vi "New Round.vi"(8 "error in (no error)":errorcluster, 10 "Move Count":i32, 11 "Grid":T1) -> (0 "error out":errorcluster, 3 "Grid out":T1)   [LabVIEW 2014, in "TeamEffort.lvclass"]
uses:
  Square/Shawn/TeamEffort/TeamEffort.lvclass
  SquareBattle Arena/Action Enum.ctl
  SquareBattle Arena/SquareBattle Arena.lvclass
  SquareBattle Arena/Direction Enum.ctl
  Player Cluster.ctl
  Grid Cluster.ctl
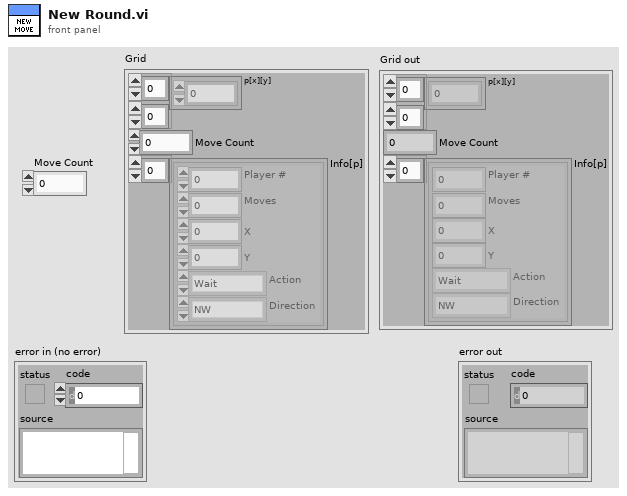
[diagram p1: front panel]
types:
  T1 = typedef "TeamEffort.lvclass/Grid Cluster.ctl" = cluster{"p[x][y]":i32[][], "Move Count":i32, "Info[p]":T2[]}
  T2 = typedef "TeamEffort.lvclass/Player Cluster.ctl" = cluster{"Player #":i32, "Moves":i32, "X":i16, "Y":i16, "Action":T3, "Direction":T4}
  T3 = typedef "SquareBattle Arena.lvlib/SquareBattle Arena.lvclass/Action Enum.ctl" = enum16{"Wait", "Move", "Attack", "Replicate"}
  T4 = typedef "SquareBattle Arena.lvlib/SquareBattle Arena.lvclass/Direction Enum.ctl" = enum16{"NW", "N", "NE", "E", "SE", "S", "SW", "W"}
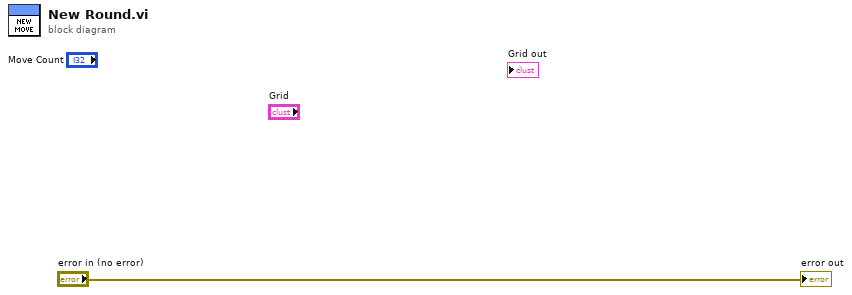
[diagram p0: block diagram]
diagram:
  "error out" <- "error in (no error)"
